vi "Brocast Data.vi"(8 "error in (no error)":errorcluster, 9 "Models Enqueue.lvclass":refnum<class "Enqueues Data.lvclass">, 10 "Views Enqueue.lvclass":refnum<class "Enqueues Data.lvclass">, 11 "MVVM Abstruct View in":refnum<class "MVVM Abstruct View.lvclass">) -> (0 "error out":errorcluster, 3 "MVVM Abstruct View out":refnum<class "MVVM Abstruct View.lvclass">)   [LabVIEW 2020, in "MMVVM Framework.lvlib" / "MVVM Abstruct View.lvlib" / "MVVM Abstruct View.lvclass"]
uses:
  MVVM Abstruct View.lvclass
  Enqueues Data/Enqueues Data.lvclass
  Enqueues Data/Enqueues Data.lvclass/Enqueues Data.ctl
  MVVM Abstruct View.lvclass/MVVM Abstruct View.ctl
  Enqueues Data/Accessors/Read ActorMap.vi
  ActorMap/ActorMap.lvclass
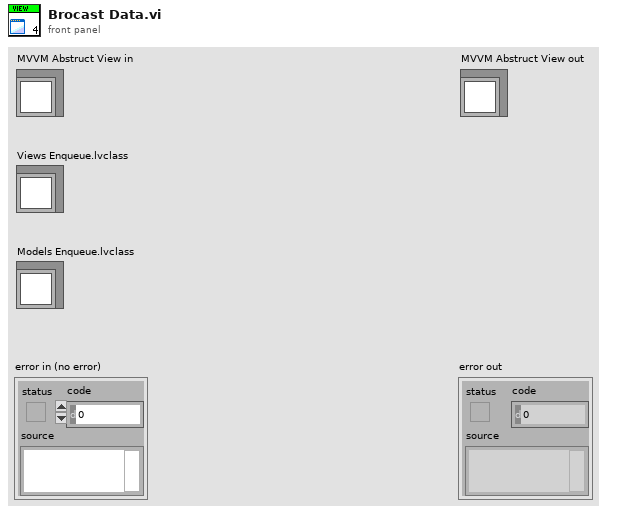
[diagram p1: front panel]
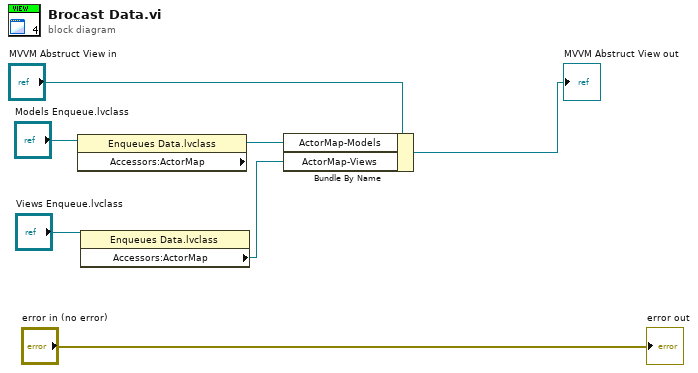
[diagram p0: block diagram]
diagram:
  n1 = property class="Enqueues Data.lvclass"(reference="Models Enqueue.lvclass") -> ("Accessors:ActorMap"=w5:refnum<class "ActorMap.lvclass">)  [unwired: 1 in, 2 out]
  n2 = property class="Enqueues Data.lvclass"(reference="Views Enqueue.lvclass") -> ("Accessors:ActorMap"=w2:refnum<class "ActorMap.lvclass">)  [unwired: 1 in, 2 out]
  n3 = Bundle By Name(cluster="MVVM Abstruct View in", "ActorMap-Models"=w5, "ActorMap-Views"=w2) -> (→"MVVM Abstruct View out":refnum<class "MVVM Abstruct View.lvclass">)
  "error out" <- "error in (no error)"
